vi "EEG_2021_099_Q2.vi"() -> ()   [LabVIEW 2022 SP3]
panel:
  out "Boolean":bool
  in  "stop":bool
  out "x":dbl
  in  "Numeric 2":dbl
  in  "Numeric":dbl
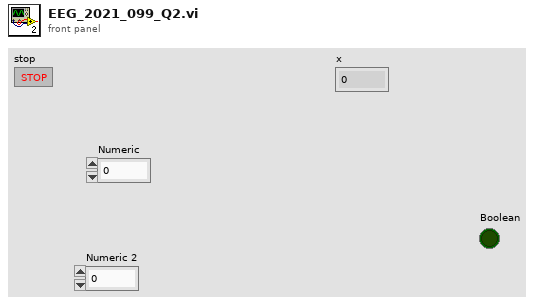
[diagram p1: front panel]
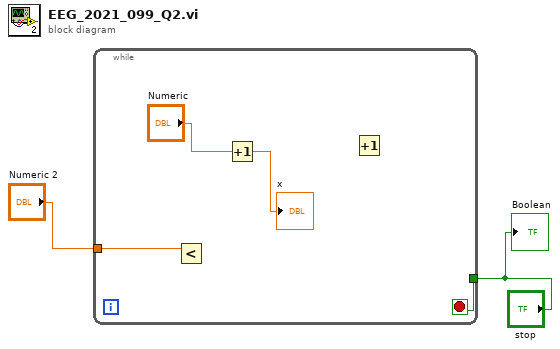
[diagram p0: block diagram]
diagram:
  n1 = while {
    tunnel: "Numeric 2" -> [w5]
    tunnel: "stop" -> [w3]
    stop <- w3 stop-if-true
    n2 = Less?(x=w5) -> ()  [unwired: 1 in, 1 out]
    n3 = Increment(x="Numeric") -> (x+1=→"x":dbl)
    n4 = Increment() -> ()  [unwired: 1 in, 1 out]
  }
  "Boolean" <- "stop"
